vi "Configure ALC Power Meter Servo.vi"(0 "VISA resource name":refnum<visa-resource-name>, 1 "Settling Error (0.2 dB)":dbl=0.2, 2 "Stop Power (1 dB)":dbl=1.0, 5 "Power Meter Channel (0: Channel A)":i32(ring) items=["Channel A", "Channel B"], 7 "Increment Percentage (100 %)":dbl=100.0, 9 "RF Output Power Limit (30 dBm)":dbl=30.0, 11 "error in (no error)":errorcluster, 12 "Start Power (0 dB)":dbl) -> (4 "VISA resource name out":refnum<visa-resource-name>, 15 "error out":errorcluster)   [LabVIEW 2018, in "Agilent PSG MXG Series.lvlib"]
doc: "Configures ALC power meter servo. \n\n<b>Note:</b>\nIt's applicable for N5171B, N5181B, N5172B, N5182B, N5173B, N5183B."
uses:
  Agilent PSG MXG Series.lvlib
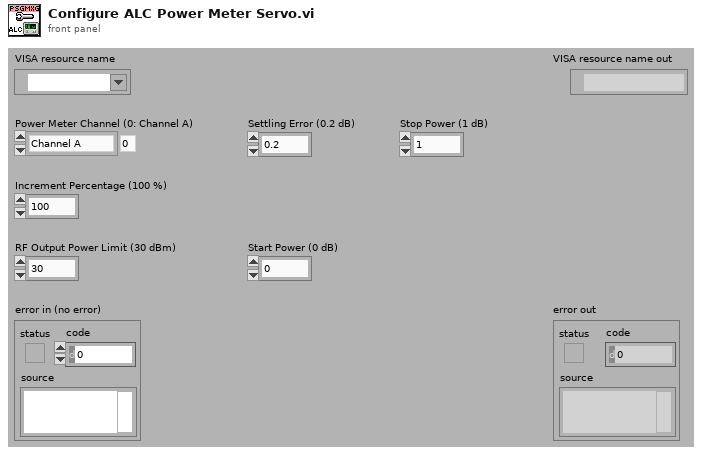
[diagram p1: front panel]
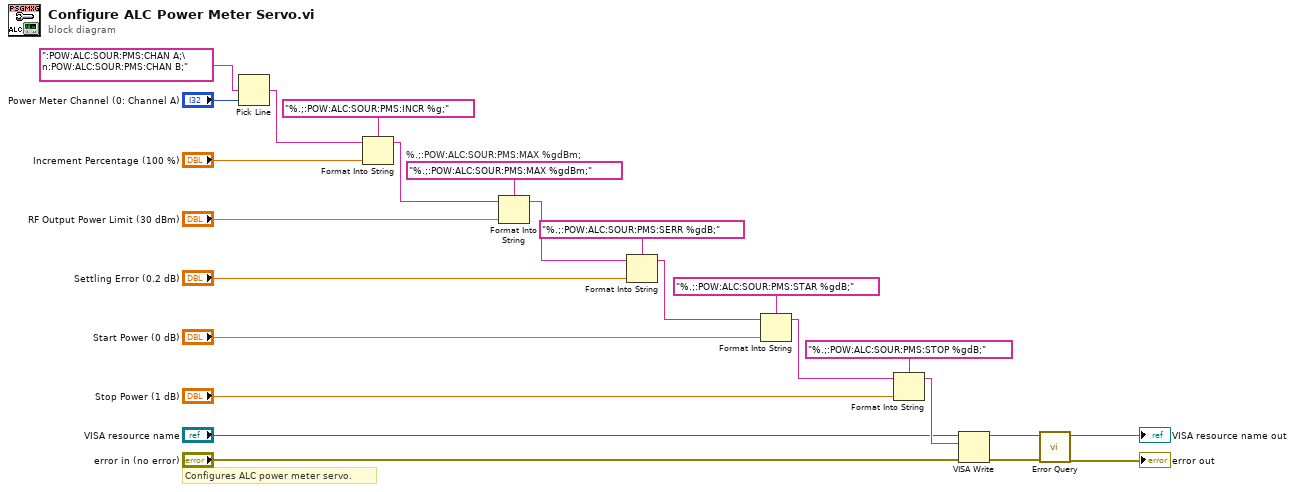
[diagram p0: block diagram]
diagram:
  w18 = "%.;:POW:ALC:SOUR:PMS:MAX %gdBm;"  # %.;:POW:ALC:SOUR:PMS:MAX %gdBm;
  # "Configures ALC power meter servo."
  n1 = Pick Line(multi-line string=":POW:ALC:SOUR:PMS:CHAN A;\n:POW:ALC:SOUR:PMS:CHAN B;", line index="Power Meter Channel (0: Channel A)") -> (output string=w22:string)  [unwired: 1 in]
  n2 = Format Into String(format string="%.;:POW:ALC:SOUR:PMS:INCR %g;", initial string=w22, "Increment Percentage (100 %)") -> (resulting string=w19:string)  [unwired: 1 in, 1 out]
  n3 = Format Into String(format string=w18, initial string=w19, "RF Output Power Limit (30 dBm)") -> (resulting string=w16:string)  [unwired: 1 in, 1 out]
  n4 = Format Into String(format string="%.;:POW:ALC:SOUR:PMS:SERR %gdB;", initial string=w16, "Settling Error (0.2 dB)") -> (resulting string=w13:string)  [unwired: 1 in, 1 out]
  n5 = Format Into String(format string="%.;:POW:ALC:SOUR:PMS:STAR %gdB;", initial string=w13, "Start Power (0 dB)") -> (resulting string=w10:string)  [unwired: 1 in, 1 out]
  n6 = Format Into String(format string="%.;:POW:ALC:SOUR:PMS:STOP %gdB;", initial string=w10, "Stop Power (1 dB)") -> (resulting string=w7:string)  [unwired: 1 in, 1 out]
  n7 = VISA Write(VISA resource name="VISA resource name", write buffer=w7, error in (no error)="error in (no error)") -> (VISA resource name out=w4:refnum<visa-resource-name>, error out=w3:errorcluster)  [unwired: 1 out]
  n8 = call "Error Query.vi"("error in (no error)"=w3, "VISA resource name"=w4) -> ("error out"=→"error out":errorcluster, "VISA resource name out"=→"VISA resource name out":refnum<visa-resource-name>)  [unwired: 6 in, 2 out]
